vi "Task Init.vi"(8 "error in (no error)":errorcluster, 11 "LoggingManager in":refnum<class "LoggingManager.lvclass">) -> (0 "error out":errorcluster, 3 "LoggingManager out":refnum<class "LoggingManager.lvclass">)   [LabVIEW 2020, in "Volatus.lvlib" / "LoggingManager.lvclass"]
uses:
  LoggingManager.lvclass
  LoggingManager.lvclass/LoggingManager.ctl
  Task/Task.lvclass
  lv-cdm/CDM-Config/Config Element/Config Element.lvclass
  C:/dev/lv20CE/relink/lv-volatus/Volatus/Task/Task.lvclass
  C:/Program Files (x86)/National Instruments/LabVIEW 2020/vi.lib/ActorFramework/Actor/Actor.lvclass
  C:/dev/lv20CE/relink/lv-volatus/Volatus/TaskStateHandler/TaskStateHandler.lvclass
  C:/dev/lv20CE/relink/lv-volatus/Volatus/VectoMessageHandler/VectoMessageHandler.lvclass
  C:/dev/lv20CE/relink/lv-volatus/Volatus/LoggingManager/LoggingManager.lvclass
  C:/dev/lv20CE/relink/lv-volatus/Volatus/API Provider/API Provider.lvclass
  C:/dev/lv20CE/relink/lv-volatus/Volatus/LoggingHandler/LoggingHandler.lvclass
  VolatusConfig/VolatusConfigElement/VolatusConfigElement.lvclass
  VolatusConfig/Task/Task.lvclass
  C:/dev/lv20CE/relink/lv-volatus/VolatusConfig/VolatusConfigElement/VolatusConfigElement.lvclass
  C:/dev/lv20CE/relink/lv-volatus/VolatusConfig/Task/Task.lvclass
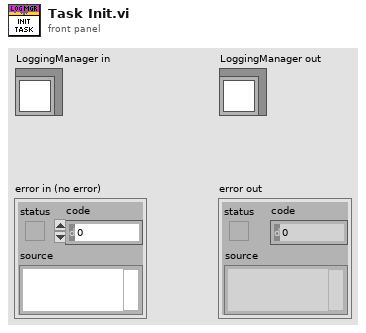
[diagram p1: front panel]
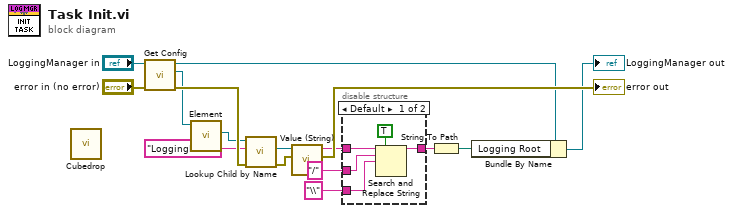
[diagram p0: block diagram]
diagram:
  n1 = call "Cubedrop.vi"() -> ()  [unwired: 12 in]
  n2 = call "Get Config.vi"("error in (no error)"="error in (no error)", "Task in"="LoggingManager in") -> ("error out"=w15:errorcluster, "Config"=w12:refnum<class "Task.lvclass">, "Task out"=w3:refnum<class "LoggingManager.lvclass">)  [unwired: 7 in]
  n3 = call "Element.vi"("VolatusConfigElement in"=w12) -> ("Element"=w11:refnum<class "Config Element.lvclass">)  [unwired: 9 in, 1 out]
  n4 = call "Lookup Child by Name.vi"("error in (no error)"=w15, "Name"="LoggingRoot", "Config Element in"=w11) -> ("error out"=w8:errorcluster, "Child"=w9:refnum<class "Config Element.lvclass">)  [unwired: 5 in, 2 out]
  n5 = call "Value (String).vi"("error in (no error)"=w8, "Config Element in"=w9) -> ("error out"=→"error out":errorcluster, "String Value"=w7:string)  [unwired: 8 in]
  n6 = disable-structure shown="Default" {
    disable-tunnel: w7 -> [w21 w22]
    disable-tunnel: "/" ("search string") -> [w20 _]
    disable-tunnel: "\\" ("search string") -> [w19 _]
    disable-tunnel: [w17 w22] -> w4
    frame condition #0 (active) {
      n7 = Search and Replace String(replace all?=TRUE ("replace all? (F)"), input string=w21, search string=w20, replace string=w19) -> (result string=w17:string)  [unwired: 4 in, 3 out]
    }
    frame condition #1 {
    }
  }
  n8 = String To Path(string=w4) -> (path=w2:path)
  n9 = Bundle By Name(cluster=w3, "Logging Root"=w2) -> (→"LoggingManager out":refnum<class "LoggingManager.lvclass">)
